vi "sys_VaribleError.vi"(9 "ErrorIn":errorcluster, 10 "Operation":enum16{"Initial", "Collect"}(ring)=enum."Collect") -> (1 "ErrorOut":errorcluster)   [LabVIEW 2013]
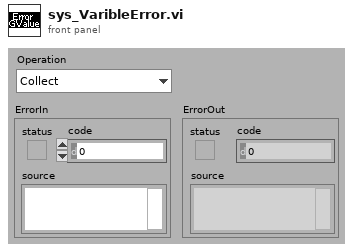
[diagram p1: front panel]
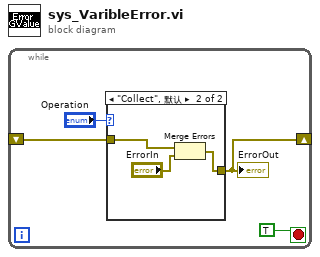
[diagram p0: block diagram]
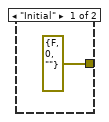
[diagram p2: hidden frame]
diagram:
  n1 = while {
    shift-right: [w1] -> _
    shift-left: _ -> [w3]
    stop <- TRUE stop-if-true
    n2 = case shown="\"Collect\", 默认" "Operation" {
      tunnel: [errorcluster {"status"=FALSE, "code"=0, "source"=""} ("error out") w7] -> w1
      tunnel: w3 -> [_ w6]
      frame "Initial" {
      }
      frame "Collect", Default {
        n3 = Merge Errors(w6, "ErrorIn") -> (w7:errorcluster)
      }
    }
    "ErrorOut" <- w1
  }
